vi "ELVIS III v1.0 Clear All IRQ.vi"(8 "error in (no error)":errorcluster) -> (0 "error out":errorcluster)   [LabVIEW 2021]
uses:
  <vilib>/myRIO/Common/Instrument Driver Framework/Utilities/typedefs/FPGA Ref Manager Action Enum.ctl
  <vilib>/myRIO/Common/Instrument Driver Framework/ELVIS III v1.0/IRQ/typedefs/ELVIS III AI IRQ Channels FPGA Reference.ctl
  <vilib>/myRIO/Common/Instrument Driver Framework/myRIO v1.0/IRQ/typedefs/Timer IRQ FPGA Reference.ctl
  <vilib>/myRIO/Common/Instrument Driver Framework/myRIO v1.0/IRQ/typedefs/DI IRQ FPGA Reference.ctl
  <vilib>/Utility/error.llb/Error Cluster From Error Code.vi
  <vilib>/rvi/errors/niLvFpgaAdjustHostInterfaceError.vi
  <vilib>/rvi/interface/nirviReadWriteControl/nirviReadWriteControl.xnode
  <vilib>/rvi/interface/Simulation/niFpgaSimulationCallBeginRW.vi
  NiFpgaLv.dll
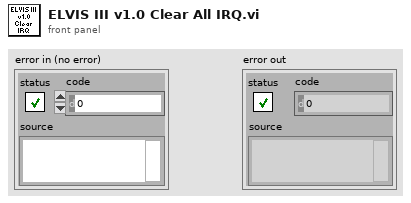
[diagram p1: front panel]
types:
  T1 = typedef "FPGA Ref Manager Action Enum.ctl" = enum16{"Get", "Set", "Reset"}
  T2 = typedef "Generic FPGA Reference.ctl" = refnum<k20>
  T3 = typedef "ELVIS III AI IRQ Channels FPGA Reference.ctl" = refnum<k20>
  T4 = typedef "Timer IRQ FPGA Reference.ctl" = refnum<k20>
  T5 = typedef "DI IRQ FPGA Reference.ctl" = refnum<k20>
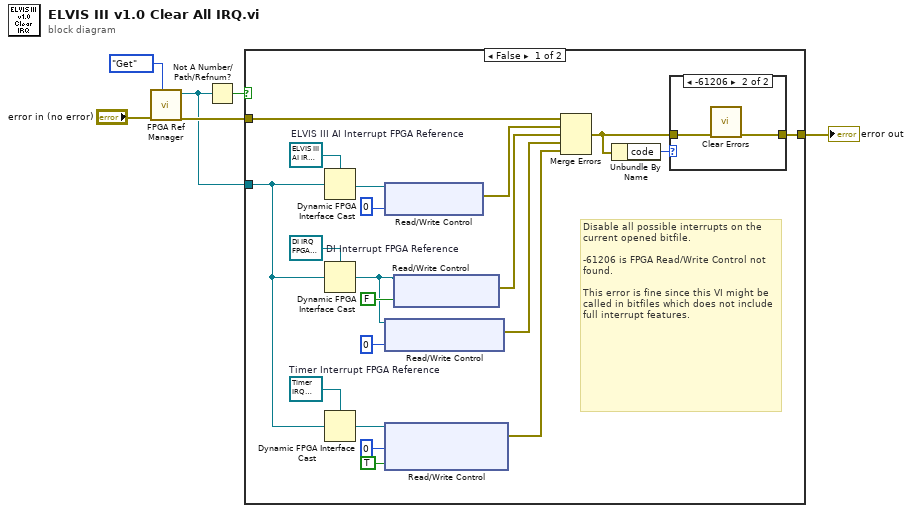
[diagram p0: block diagram]
diagram:
  n1 = call <vilib>:"FPGA Ref Manager.vi"("Action"=FPGA_Ref_Manager_Action_Enum."Get", "error in (no error)"="error in (no error)") -> ("error out"=w3:errorcluster, "Generic FPGA Reference out"=w2:T2)  [unwired: 7 in]
  n2 = Not A Number/Path/Refnum?(number/path/refnum=w2) -> (NaN/Path/Refnum?=w1:bool)
  n3 = case shown="False" w1 {
    tunnel: [w20 w30] -> w4
    tunnel: w2 -> [w24 _]
    tunnel: w3 -> [w23 w30]
    frame False {
      w14 = T3 refnum  # ELVIS III AI Interrupt FPGA Reference
      w25 = T4 refnum  # Timer Interrupt FPGA Reference
      w26 = T5 refnum  # DI Interrupt FPGA Reference
      # "Disable all possible interrupts on the current opened bitfile.\n\n-61206 is FPGA Read/Write Control not found.\n\nThis error is fine since this VI might be called in bitfiles which does not include full interrupt features."
      n4 = Dynamic FPGA Interface Cast(Session In=w14, Type=w24) -> (Session Out=w13:T3)
      n5 = Dynamic FPGA Interface Cast(Session In=w26, Type=w24) -> (Session Out=w10:T5)
      n6 = Dynamic FPGA Interface Cast(Session In=w25, Type=w24) -> (Session Out=w18:T4)
      n7 = xnode "Read/Write Control"("FPGA VI Reference In"=w13, "IRQ.AI_A.CNFG"=u8 0 ("AI.A.IRQ.CNFG")) -> ("error out"=w15:errorcluster)  [unwired: 1 in, 1 out]
      n8 = xnode "Read/Write Control"("FPGA VI Reference In"=w10, "IRQ.DIO_A_7:0.ENA"=u8 0 ("DIO.A_7:0.IRQ.ENA")) -> ("error out"=w9:errorcluster)  [unwired: 1 in, 1 out]
      n9 = xnode "Read/Write Control"("FPGA VI Reference In"=w18, "IRQ.TIMER.WRITE"=u32 0 ("Timeout"), "IRQ.TIMER.SETTIME"=TRUE ("TIMER.SetTime")) -> ("error out"=w8:errorcluster)  [unwired: 1 in, 1 out]
      n10 = xnode "Read/Write Control"("FPGA VI Reference In"=w10, "IRQ.DI_BTN.ENA"=FALSE ("DI.BTN.IRQ.ENA")) -> ("error out"=w7:errorcluster)  [unwired: 1 in, 1 out]
      n11 = Merge Errors(w23, w15, w7, w9, w8) -> (w21:errorcluster)
      n12 = Unbundle By Name(w21) -> ("code"=w22:i32)
      n13 = case shown="-61206" w22 {
        tunnel: [w27 w28] -> w20
        tunnel: w21 -> [w27 w29]
        frame Default {
        }
        frame -61206 {
          n14 = call <vilib>:"Clear Errors.vi"("error in (no error)"=w29) -> ("error out"=w28:errorcluster)  [unwired: 5 in, 1 out]
        }
      }
    }
    frame True {
    }
  }
  "error out" <- w4
